vi "Initialise.vi"(8 "error in (no error)":errorcluster, 10 "Request Channel":refnum<class "Messenger.lvclass">, 11 "Actor API in":refnum<class "Actor API.lvclass">) -> (0 "error out":errorcluster, 3 "Actor API out":refnum<class "Actor API.lvclass">)   [LabVIEW 2015, in "Actor API.lvclass"]
uses:
  Actor API.lvclass
  Messaging/Messenger/Messenger.lvclass
  Actor API.lvclass/Actor API.ctl
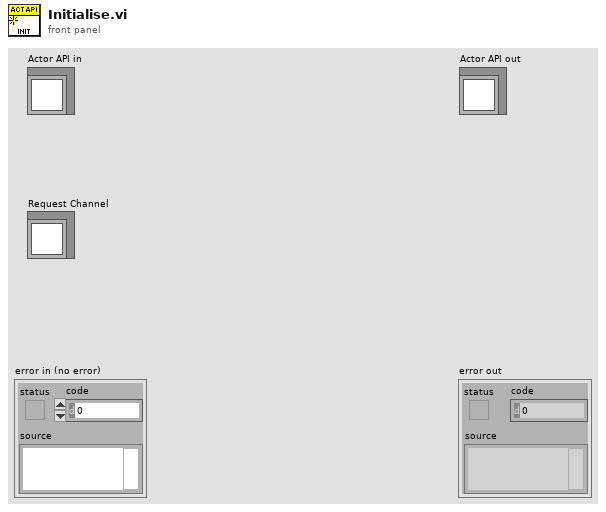
[diagram p1: front panel]
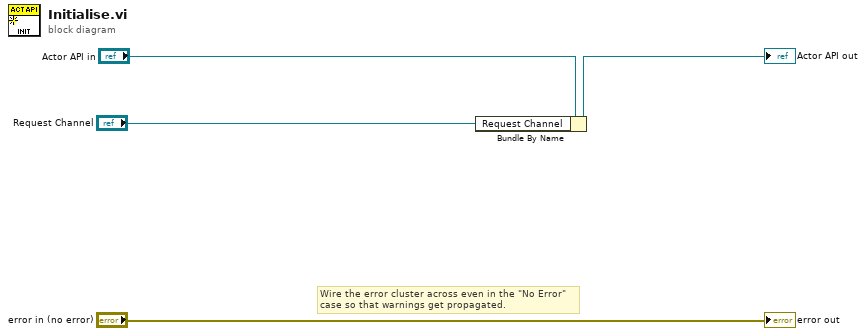
[diagram p0: block diagram]
diagram:
  # "Wire the error cluster across even in the \"No Error\"\ncase so that warnings get propagated."
  n1 = Bundle By Name(cluster="Actor API in", "Request Channel"="Request Channel") -> (→"Actor API out":refnum<class "Actor API.lvclass">)
  "error out" <- "error in (no error)"
